vi "LV SciSDK REGISTER FILE GET REGISTER.vi"(8 "error in (no error)":errorcluster, 9 "Register File Handle In":T1, 10 "Register Name":string) -> (0 "error out":errorcluster, 1 "Register File Handle Out":T1, 11 "Value":i32)   [LabVIEW 2021]
uses:
  SciSDK_Labview.lvlib
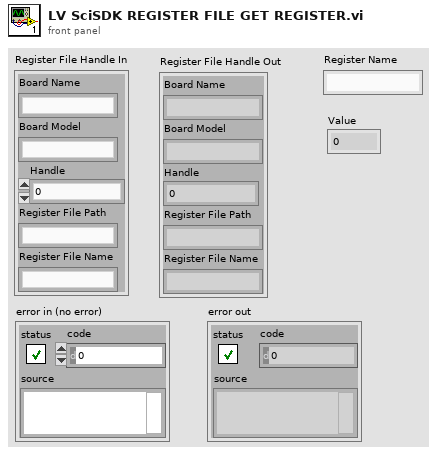
[diagram p1: front panel]
types:
  T1 = cluster{"Board Name":string, "Board Model":string, "Handle":u64, "Register File Path":string, "Register File Name":string}
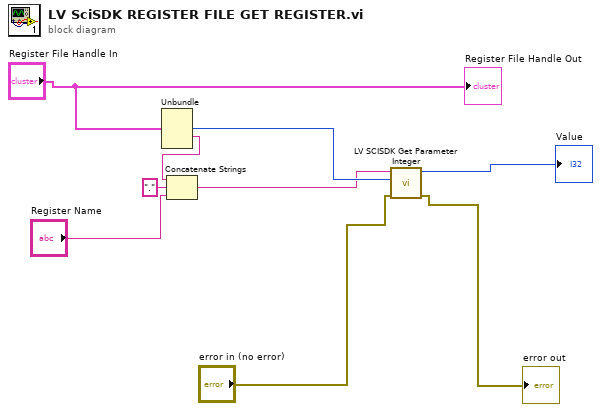
[diagram p0: block diagram]
diagram:
  n1 = Unbundle("Register File Handle In") -> ("Handle"=w5:u64, "Register File Path"=w8:string)  [unwired: 3 out]
  n2 = Concatenate Strings(w8, "." ("string"), "Register Name") -> (w4:string)
  n3 = call "LV SCISDK Get Parameter Integer.vi"("error in (no error)"="error in (no error)", "handle"=w5, "Path"=w4) -> ("error out"=→"error out":errorcluster, "value"=→"Value":i32)  [unwired: 5 in, 2 out]
  "Register File Handle Out" <- "Register File Handle In"
